vi "Generate Configuration.vi"(6 "Starting Address Offset":u16 format="%04x", 7 "Virtual Memory Unit in":refnum<class "Virtual Memory Unit.lvclass">, 8 "error in (no error)":errorcluster, 11 "Remote Terminal in":refnum<class "Remote Terminal.lvclass">) -> (0 "error out":errorcluster, 2 "Parameter List":string[](array[string]), 3 "Remote Terminal out":refnum<class "Remote Terminal.lvclass">, 4 "Next Address Offset":u16 format="%04x", 5 "Virtual Memory Unit out":refnum<class "Virtual Memory Unit.lvclass">)   [LabVIEW 2020, in "BCI-1553 API.lvlib" / "Remote Terminal.lvclass"]
doc: "Generates the entire configuration for this Remote Terminal. Does not push it to the 1553 Session component yet."
uses:
  Remote Terminal.lvclass
  C:/Users/MattJ/Desktop/git/bci-1553-labview-api/src/1553 SubComponent/1553 SubComponent.lvclass
  Dependencies/Virtual Memory Unit/Virtual Memory Unit.lvclass
  Dependencies/Registry/Registry.lvclass/Registry.ctl
  Dependencies/Registry/Registry.lvclass
  1553 SubComponent/1553 SubComponent.lvclass
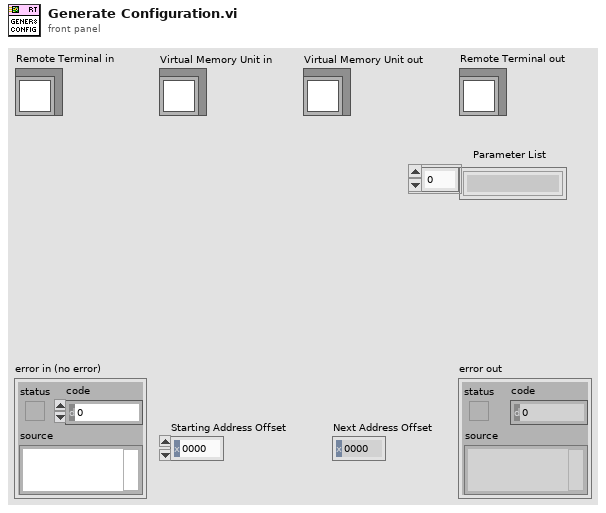
[diagram p1: front panel]
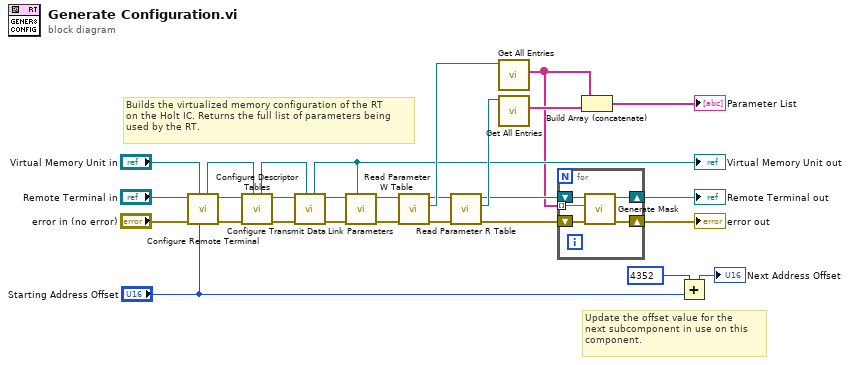
[diagram p0: block diagram]
diagram:
  # "Update the offset value for the\nnext subcomponent in use on this\ncomponent."
  # "Builds the virtualized memory configuration of the RT\non the Holt IC. Returns the full list of parameters being\nused by the RT."
  n1 = call "Configure Remote Terminal.vi"("Starting Address Offset"="Starting Address Offset", "Virtual Memory Unit in"="Virtual Memory Unit in", "error in (no error)"="error in (no error)", "Remote Terminal in"="Remote Terminal in") -> ("error out"=w25:errorcluster, "Remote Terminal out"=w26:refnum<class "Remote Terminal.lvclass">, "Virtual Memory Unit out"=w19:refnum<class "Virtual Memory Unit.lvclass">)  [unwired: 5 in]
  n2 = call "Configure Descriptor Tables.vi"("Virtual Memory Unit in"=w19, "error in (no error)"=w25, "Remote Terminal in"=w26) -> ("error out"=w23:errorcluster, "Remote Terminal out"=w24:refnum<class "Remote Terminal.lvclass">, "Virtual Memory Unit out"=w18:refnum<class "Virtual Memory Unit.lvclass">)  [unwired: 6 in]
  n3 = call "Configure Transmit Data.vi"("Virtual Memory Unit in"=w18, "error in (no error)"=w23, "Remote Terminal in"=w24) -> ("error out"=w21:errorcluster, "Remote Terminal out"=w22:refnum<class "Remote Terminal.lvclass">, "Virtual Memory Unit out"=w11:refnum<class "Virtual Memory Unit.lvclass">)  [unwired: 6 in]
  "Virtual Memory Unit out" <- w11
  n4 = call "Link Parameters.vi"("Virtual Memory Unit in"=w11, "error in (no error)"=w21, "Remote Terminal in"=w22) -> ("error out"=w16:errorcluster, "Remote Terminal out"=w10:refnum<class "Remote Terminal.lvclass">)  [unwired: 7 in]
  n5 = call-dynamic "Read Parameter W Table.vi"("error in (no error)"=w16, "1553 SubComponent in"=w10) -> ("error out"=w17:errorcluster, "Parameter W Table"=w15:refnum<class "Registry.lvclass">, "1553 SubComponent out"=w9:refnum<class "Remote Terminal.lvclass">)  [unwired: 7 in]
  n6 = call-dynamic "Read Parameter R Table.vi"("error in (no error)"=w17, "1553 SubComponent in"=w9) -> ("error out"=w8:errorcluster, "Parameter R Table"=w14:refnum<class "Registry.lvclass">, "1553 SubComponent out"=w7:refnum<class "Remote Terminal.lvclass">)  [unwired: 7 in]
  n7 = call "Get All Entries.vi"("Registry in"=w15) -> ("Keys"=w6:string[])  [unwired: 8 in, 2 out]
  n8 = call "Get All Entries.vi"("Registry in"=w14) -> ("Keys"=w13:string[])  [unwired: 8 in, 2 out]
  n9 = for {
    tunnel: w6 -> [w31] mode=indexing
    shift-right: [w29] -> w4
    shift-left: w7 -> [w32]
    shift-right: [w30] -> w5
    shift-left: w8 -> [w33]
    n10 = call "Generate Mask.vi"("error in (no error)"=w33, "Parameter"=w31, "1553 SubComponent in"=w32) -> ("error out"=w30:errorcluster, "1553 SubComponent out"=w29:refnum<class "Remote Terminal.lvclass">)  [unwired: 7 in]
  }
  "error out" <- w5
  "Remote Terminal out" <- w4
  n11 = Build Array (concatenate)(w6, w13) -> (→"Parameter List":string[])
  n12 = Add(x=u16 4352 ("Address"), y="Starting Address Offset") -> (x+y=→"Next Address Offset":u16)
